vi "Test command line.vi"() -> ()   [LabVIEW 2014]
panel:
  in  "command line":string="ls"
  out "standard output":string
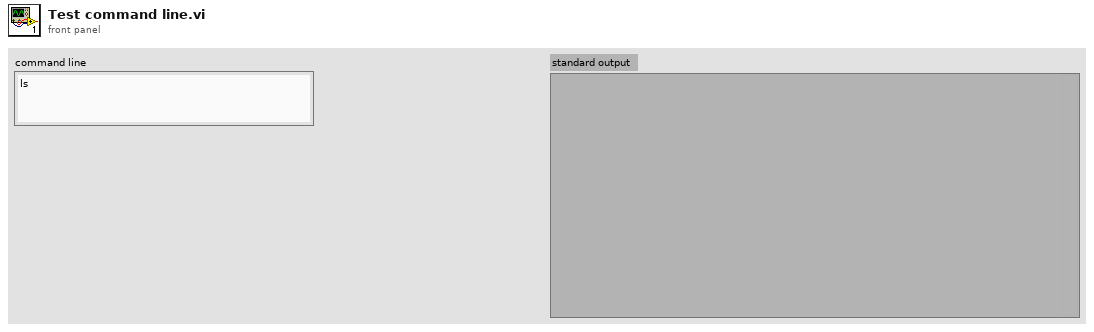
[diagram p1: front panel]
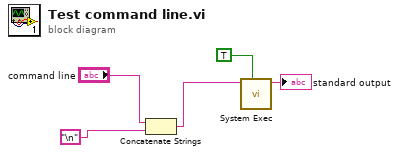
[diagram p0: block diagram]
diagram:
  n1 = Concatenate Strings("command line", "\n") -> (w1:string)
  n2 = call <vilib>:"System Exec.vi"("wait until completion? (T)"=TRUE, "command line"=w1) -> ("standard output"=→"standard output":string)  [unwired: 6 in, 3 out]
